vi "Process Data.vi"(7 "AdasLvTemplate in":refnum<class "AdasLvTemplate.lvclass">, 8 "error in":errorcluster, 11 "Node in":refnum<class "ThermotronDriver.lvclass">) -> (0 "error out":errorcluster, 3 "Node out":refnum<class "ThermotronDriver.lvclass">, 5 "AdasLvTemplate out":refnum<class "AdasLvTemplate.lvclass">)   [LabVIEW 2023, in "ThermotronDriver.lvlib" / "ThermotronDriver.lvclass"]
uses:
  ThermotronDriver.lvclass
  <vilib>/ADAS Replay HIL/ADAS Plugin Utilities/AdasLvTemplate/AdasLvTemplate.lvclass
  ThermotronDriver.lvclass/ThermotronDriver.ctl
  <vilib>/ADAS Replay HIL/ADAS Plugin Utilities/AdasLvTemplate/Typedefs/Out Of Band/Status Custom DBL Selector.ctl
  <vilib>/ADAS Replay HIL/ADAS Plugin Utilities/AdasLvTemplate/AdasLvTemplate.lvclass/AdasLvTemplate.ctl
  Support/LabVIEW API/Thermotron8800InstrumentDriver64bitForLabView2018/Thermotron 8800/Thermotron 8800.lvlib
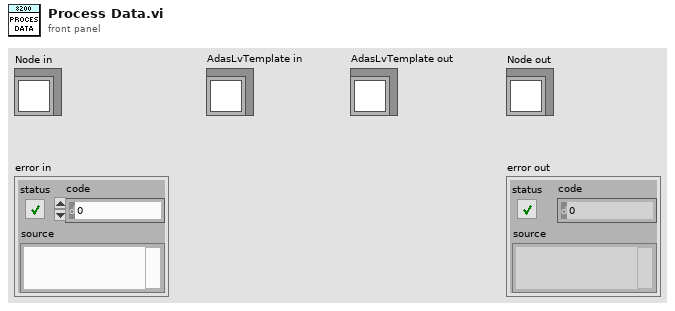
[diagram p1: front panel]
types:
  T1 = typedef "AdasLvTemplate.lvlib/AdasLvTemplate.lvclass/Status Custom DBL Selector.ctl" = enum16{"Custom 5 (DBL)", "Custom 6 (DBL)", "Custom 7 (DBL)", "Custom 8 (DBL)"}
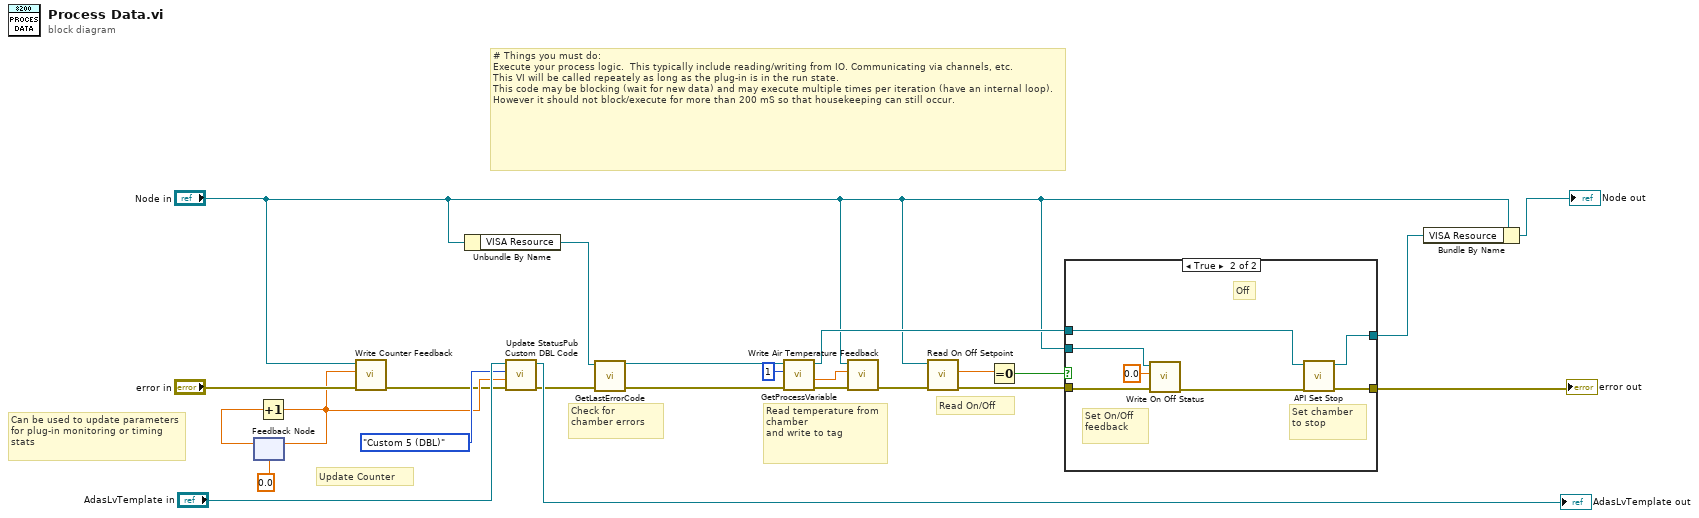
[diagram p0: block diagram]
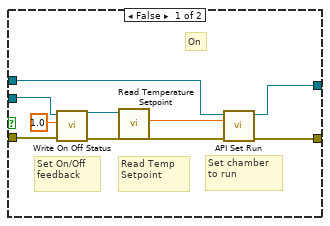
[diagram p2: hidden frame]
diagram:
  # "Update Counter"
  # "Read On/Off"
  # "Read temperature from chamber\nand write to tag"
  # "Check for\nchamber errors"
  # "# Things you must do:\nExecute your process logic.  This typically include reading/writing from IO. Communicating via channels, etc.  \nThis VI will be called repeately as long as the plug-in is in the run state.\nThis code may be blocking (wait for new data) and may execute multiple times per iteration (have an internal loop).  However it should not block/execute for more than 200 mS so that housekeeping can still occur."
  # "Can be used to update parameters for plug-in monitoring or timing stats"
  n1 = feedback #1(0.0) -> (w24:dbl)
  n2 = Increment(x=w24) -> (x+1=w18:dbl)
  n3 = feedback-in #1(w18) -> ()
  n4 = call-dynamic "Write Counter Feedback.vi"("error in (no error)"="error in", "Counter"=w18, "ThermotronDriver in"="Node in") -> ("error out"=w17:errorcluster)  [unwired: 7 in, 1 out]
  n5 = Unbundle By Name("Node in") -> ("VISA Resource"=w5:refnum<visa-resource-name>)
  n6 = call <vilib>:"Update StatusPub Custom DBL Code.vi"("error in (no error)"=w17, "Custom Data"=w18, "Terminal"=Status_Custom_DBL_Selector."Custom 5 (DBL)", "AdasLvTemplate in"="AdasLvTemplate in") -> ("error out"=w13:errorcluster, "AdasLvTemplate out"=→"AdasLvTemplate out":refnum<class "AdasLvTemplate.lvclass">)  [unwired: 6 in]
  n7 = call "GetLastErrorCode.vi"("error in"=w13, "VISA resource name"=w5) -> ("error out"=w12:errorcluster, "VISA resource name out"=w11:refnum<visa-resource-name>)  [unwired: 6 in, 2 out]
  n8 = call "GetProcessVariable.vi"("error in"=w12, "Channel (1-140)"=u16 1, "VISA resource name"=w11) -> ("error out"=w15:errorcluster, "Process Variable"=w14:dbl, "VISA resource name out"=w4:refnum<visa-resource-name>)  [unwired: 5 in, 1 out]
  n9 = call-dynamic "Write Air Temperature Feedback.vi"("error in (no error)"=w15, "Temperature Feedback"=w14, "ThermotronDriver in"="Node in") -> ("error out"=w10:errorcluster)  [unwired: 7 in, 1 out]
  n10 = call-dynamic "Read On Off Setpoint.vi"("error in (no error)"=w10, "ThermotronDriver in"="Node in") -> ("error out"=w7:errorcluster, "On Off Setpoint"=w9:dbl)  [unwired: 7 in, 1 out]
  n11 = Equal To 0?(x=w9) -> (x = 0?=w8:bool)
  n12 = case shown="True" w8 {
    tunnel: w7 -> [w34 w40]
    tunnel: "Node in" -> [w33 w39]
    tunnel: [w31 w37] -> w6
    tunnel: w4 -> [w30 w36]
    tunnel: [w29 w35] -> w2
    frame False {
      # "Read Temp\nSetpoint"
      # "Set chamber\nto run"
      # "Set On/Off\nfeedback"
      # "On"
      n13 = call-dynamic "Write On Off Status.vi"("error in (no error)"=w34, "On Off Status"=1.0, "ThermotronDriver in"=w33) -> ("error out"=w27:errorcluster, "ThermotronDriver out"=w28:refnum<class "ThermotronDriver.lvclass">)  [unwired: 7 in]
      n14 = call-dynamic "Read Temperature Setpoint.vi"("error in (no error)"=w27, "ThermotronDriver in"=w28) -> ("error out"=w25:errorcluster, "Temperature Setpoint"=w26:dbl)  [unwired: 7 in, 1 out]
      n15 = call "API Set Run.vi"("error in"=w25, "Air Temperature Setpoint"=w26, "VISA resource name"=w30) -> ("error out"=w31:errorcluster, "VISA resource name out"=w29:refnum<visa-resource-name>)  [unwired: 7 in]
    }
    frame True {
      # "Set chamber\nto stop"
      # "Set On/Off\nfeedback"
      # "Off"
      n16 = call-dynamic "Write On Off Status.vi"("error in (no error)"=w40, "On Off Status"=0.0, "ThermotronDriver in"=w39) -> ("error out"=w38:errorcluster)  [unwired: 7 in, 1 out]
      n17 = call "API Set Stop.vi"("error in"=w38, "VISA resource name"=w36) -> ("error out"=w37:errorcluster, "VISA resource name out"=w35:refnum<visa-resource-name>)  [unwired: 8 in]
    }
  }
  "error out" <- w6
  n18 = Bundle By Name(cluster="Node in", "VISA Resource"=w2) -> (→"Node out":refnum<class "ThermotronDriver.lvclass">)
